vi "crane_anim_init.vi"() -> (1 "Trolley":refnum<vi>, 4 "Main":refnum<vi>(3d-picture), 5 "Pivot Beta":refnum<vi>, 6 "Arm":refnum<vi>, 7 "Load":refnum<vi>, 8 "Target":refnum<vi>, 9 "Load Line":refnum<vi>, 10 "Pivot Alpha":refnum<vi>)   [LabVIEW 2009]
uses:
  <vilib>/picture/3D Picture Control/NI_3D Picture Control.lvlib
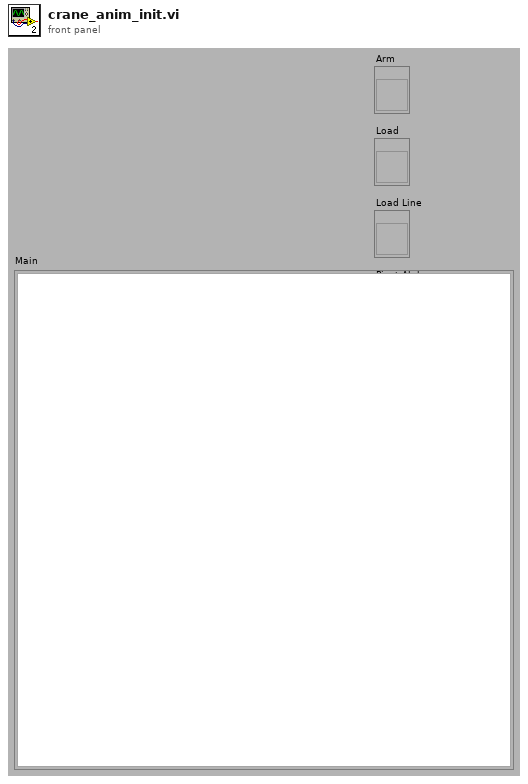
[diagram p1: front panel]
types:
  T1 = cluster{"Red":sgl, "Green":sgl, "Blue":sgl, "Alpha":sgl}
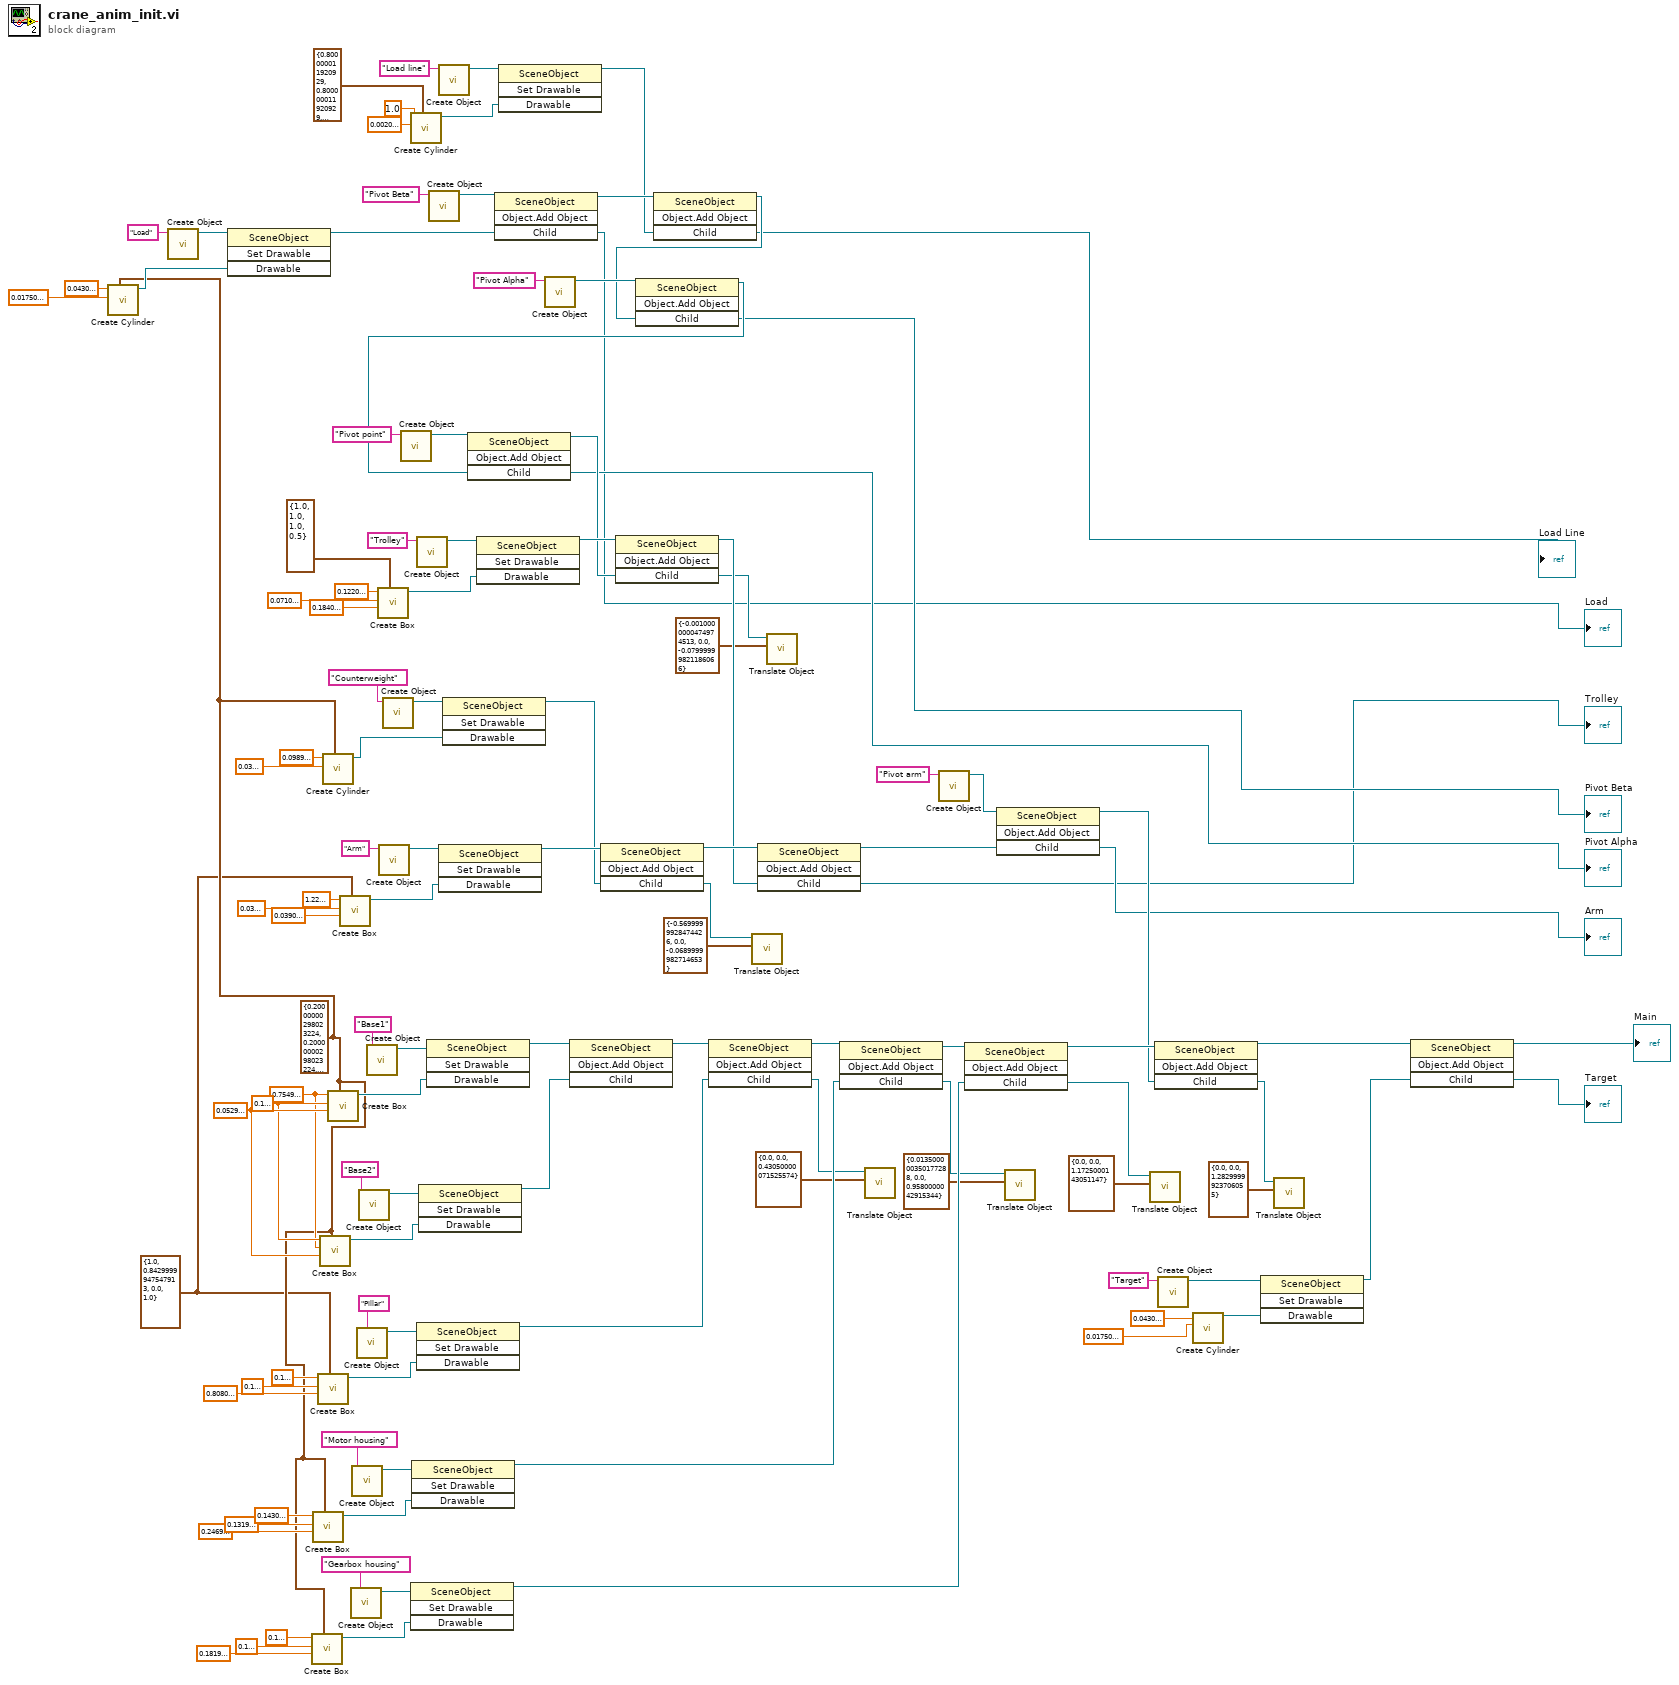
[diagram p0: block diagram]
diagram:
  w21 = T1 {"Red"=1.0, "Green"=0.843, "Blue"=0.0, "Alpha"=1.0} ("Color")
  w111 = sgl 0.053 ("Length Z")
  w110 = sgl 0.1 ("Length Y")
  w109 = sgl 0.755 ("Length X")
  w22 = T1 {"Red"=0.2, "Green"=0.2, "Blue"=0.2, "Alpha"=1.0} ("Color")
  n1 = call <vilib>:"Create Cylinder.vi"("Color"=w22, "Radius"=sgl 0.0175, "Height"=sgl 0.043) -> ("New Cylinder Refnum"=w57:refnum<vi>)  [unwired: 7 in, 1 out]
  n2 = call <vilib>:"Create Object.vi"("Name"="Load") -> ("Scene:New Object"=w58:refnum<vi>)  [unwired: 9 in, 1 out]
  n3 = invoke class="SceneObject" method="Set Drawable"(reference=w58, "Drawable"=w57) -> (reference out=w37:refnum<vi>)  [unwired: 2 in, 3 out]
  n4 = call <vilib>:"Create Box.vi"("Color"=w22, "Length Z"=sgl 0.182, "Length Y"=sgl 0.1, "Length X"=sgl 0.1) -> ("New Box Refnum"=w95:refnum<vi>)  [unwired: 6 in, 1 out]
  n5 = call <vilib>:"Create Box.vi"("Color"=w22, "Length Z"=sgl 0.247, "Length Y"=sgl 0.132, "Length X"=sgl 0.143) -> ("New Box Refnum"=w100:refnum<vi>)  [unwired: 6 in, 1 out]
  n6 = call <vilib>:"Create Box.vi"("Color"=w21, "Length Z"=sgl 0.808, "Length Y"=sgl 0.1, "Length X"=sgl 0.1) -> ("New Box Refnum"=w105:refnum<vi>)  [unwired: 6 in, 1 out]
  n7 = call <vilib>:"Create Box.vi"("Color"=w22, "Length Z"=w111, "Length Y"=w109, "Length X"=w110) -> ("New Box Refnum"=w112:refnum<vi>)  [unwired: 6 in, 1 out]
  n8 = call <vilib>:"Create Cylinder.vi"("Color"=w22, "Radius"=sgl 0.04, "Height"=sgl 0.099) -> ("New Cylinder Refnum"=w71:refnum<vi>)  [unwired: 7 in, 1 out]
  n9 = call <vilib>:"Create Box.vi"("Color"=w22, "Length Z"=w111, "Length Y"=w110, "Length X"=w109) -> ("New Box Refnum"=w114:refnum<vi>)  [unwired: 6 in, 1 out]
  n10 = call <vilib>:"Create Box.vi"("Color"=w21, "Length Z"=sgl 0.039, "Length Y"=sgl 0.04, "Length X"=sgl 1.22) -> ("New Box Refnum"=w78:refnum<vi>)  [unwired: 6 in, 1 out]
  n11 = call <vilib>:"Create Object.vi"("Name"="Gearbox housing") -> ("Scene:New Object"=w96:refnum<vi>)  [unwired: 9 in, 1 out]
  n12 = call <vilib>:"Create Object.vi"("Name"="Motor housing") -> ("Scene:New Object"=w101:refnum<vi>)  [unwired: 9 in, 1 out]
  n13 = call <vilib>:"Create Object.vi"("Name"="Pillar") -> ("Scene:New Object"=w106:refnum<vi>)  [unwired: 9 in, 1 out]
  n14 = call <vilib>:"Create Object.vi"("Name"="Base2") -> ("Scene:New Object"=w113:refnum<vi>)  [unwired: 9 in, 1 out]
  n15 = call <vilib>:"Create Object.vi"("Name"="Base1") -> ("Scene:New Object"=w115:refnum<vi>)  [unwired: 9 in, 1 out]
  n16 = call <vilib>:"Create Box.vi"("Color"=T1 {"Red"=1.0, "Green"=1.0, "Blue"=1.0, "Alpha"=0.5}, "Length Z"=sgl 0.184, "Length Y"=sgl 0.071, "Length X"=sgl 0.122) -> ("New Box Refnum"=w62:refnum<vi>)  [unwired: 6 in, 1 out]
  n17 = call <vilib>:"Create Object.vi"("Name"="Arm") -> ("Scene:New Object"=w79:refnum<vi>)  [unwired: 9 in, 1 out]
  n18 = call <vilib>:"Create Object.vi"("Name"="Counterweight") -> ("Scene:New Object"=w72:refnum<vi>)  [unwired: 9 in, 1 out]
  n19 = call <vilib>:"Create Object.vi"("Name"="Pivot point") -> ("Scene:New Object"=w34:refnum<vi>)  [unwired: 9 in, 1 out]
  n20 = call <vilib>:"Create Cylinder.vi"("Color"=T1 {"Red"=0.8, "Green"=0.8, "Blue"=0.8, "Alpha"=1.0}, "Radius"=sgl 0.002, "Height"=sgl 1.0) -> ("New Cylinder Refnum"=w14:refnum<vi>)  [unwired: 7 in, 1 out]
  n21 = invoke class="SceneObject" method="Set Drawable"(reference=w96, "Drawable"=w95) -> (reference out=w86:refnum<vi>)  [unwired: 2 in, 3 out]
  n22 = invoke class="SceneObject" method="Set Drawable"(reference=w101, "Drawable"=w100) -> (reference out=w88:refnum<vi>)  [unwired: 2 in, 3 out]
  n23 = call <vilib>:"Create Object.vi"("Name"="Trolley") -> ("Scene:New Object"=w63:refnum<vi>)  [unwired: 9 in, 1 out]
  n24 = invoke class="SceneObject" method="Set Drawable"(reference=w106, "Drawable"=w105) -> (reference out=w89:refnum<vi>)  [unwired: 2 in, 3 out]
  n25 = invoke class="SceneObject" method="Set Drawable"(reference=w113, "Drawable"=w112) -> (reference out=w107:refnum<vi>)  [unwired: 2 in, 3 out]
  n26 = invoke class="SceneObject" method="Set Drawable"(reference=w115, "Drawable"=w114) -> (reference out=w108:refnum<vi>)  [unwired: 2 in, 3 out]
  n27 = call <vilib>:"Create Object.vi"("Name"="Pivot Beta") -> ("Scene:New Object"=w39:refnum<vi>)  [unwired: 9 in, 1 out]
  n28 = call <vilib>:"Create Object.vi"("Name"="Load line") -> ("Scene:New Object"=w16:refnum<vi>)  [unwired: 9 in, 1 out]
  n29 = invoke class="SceneObject" method="Set Drawable"(reference=w79, "Drawable"=w78) -> (reference out=w68:refnum<vi>)  [unwired: 2 in, 3 out]
  n30 = invoke class="SceneObject" method="Set Drawable"(reference=w72, "Drawable"=w71) -> (reference out=w67:refnum<vi>)  [unwired: 2 in, 3 out]
  n31 = invoke class="SceneObject" method="Set Drawable"(reference=w63, "Drawable"=w62) -> (reference out=w53:refnum<vi>)  [unwired: 2 in, 3 out]
  n32 = invoke class="SceneObject" method="Object.Add Object"(reference=w39, "Child"=w37) -> (reference out=w19:refnum<vi>, "Child"=→"Load":refnum<vi>)  [unwired: 2 in, 2 out]
  n33 = invoke class="SceneObject" method="Set Drawable"(reference=w16, "Drawable"=w14) -> (reference out=w17:refnum<vi>)  [unwired: 2 in, 3 out]
  n34 = call <vilib>:"Create Object.vi"("Name"="Pivot Alpha") -> ("Scene:New Object"=w52:refnum<vi>)  [unwired: 9 in, 1 out]
  n35 = invoke class="SceneObject" method="Object.Add Object"(reference=w108, "Child"=w107) -> (reference out=w91:refnum<vi>)  [unwired: 2 in, 3 out]
  n36 = invoke class="SceneObject" method="Object.Add Object"(reference=w68, "Child"=w67) -> (reference out=w64:refnum<vi>, "Child"=w66:refnum<vi>)  [unwired: 2 in, 2 out]
  n37 = invoke class="SceneObject" method="Object.Add Object"(reference=w19, "Child"=w17) -> (reference out=w18:refnum<vi>, "Child"=→"Load Line":refnum<vi>)  [unwired: 2 in, 2 out]
  n38 = invoke class="SceneObject" method="Object.Add Object"(reference=w52, "Child"=w18) -> (reference out=w35:refnum<vi>, "Child"=→"Pivot Beta":refnum<vi>)  [unwired: 2 in, 2 out]
  n39 = invoke class="SceneObject" method="Object.Add Object"(reference=w34, "Child"=w35) -> (reference out=w36:refnum<vi>, "Child"=→"Pivot Alpha":refnum<vi>)  [unwired: 2 in, 2 out]
  n40 = invoke class="SceneObject" method="Object.Add Object"(reference=w53, "Child"=w36) -> (reference out=w54:refnum<vi>, "Child"=w50:refnum<vi>)  [unwired: 2 in, 2 out]
  n41 = invoke class="SceneObject" method="Object.Add Object"(reference=w91, "Child"=w89) -> (reference out=w90:refnum<vi>, "Child"=w85:refnum<vi>)  [unwired: 2 in, 2 out]
  n42 = call <vilib>:"Translate Object.vi"("Translation"=cluster{"X":sgl, "Y":sgl, "Z":sgl} {"X"=-0.57, "Y"=0.0, "Z"=-0.069}, "Scene.Object In"=w66) -> ()  [unwired: 8 in, 2 out]
  n43 = invoke class="SceneObject" method="Object.Add Object"(reference=w64, "Child"=w54) -> (reference out=w30:refnum<vi>, "Child"=→"Trolley":refnum<vi>)  [unwired: 2 in, 2 out]
  n44 = call <vilib>:"Translate Object.vi"("Translation"=cluster{"X":sgl, "Y":sgl, "Z":sgl} {"X"=-0.001, "Y"=0.0, "Z"=-0.08}, "Scene.Object In"=w50) -> ()  [unwired: 8 in, 2 out]
  n45 = invoke class="SceneObject" method="Object.Add Object"(reference=w90, "Child"=w88) -> (reference out=w87:refnum<vi>, "Child"=w83:refnum<vi>)  [unwired: 2 in, 2 out]
  n46 = call <vilib>:"Translate Object.vi"("Translation"=cluster{"X":sgl, "Y":sgl, "Z":sgl} {"X"=0.0, "Y"=0.0, "Z"=0.4305}, "Scene.Object In"=w85) -> ()  [unwired: 8 in, 2 out]
  n47 = call <vilib>:"Create Object.vi"("Name"="Pivot arm") -> ("Scene:New Object"=w32:refnum<vi>)  [unwired: 9 in, 1 out]
  n48 = invoke class="SceneObject" method="Object.Add Object"(reference=w87, "Child"=w86) -> (reference out=w74:refnum<vi>, "Child"=w81:refnum<vi>)  [unwired: 2 in, 2 out]
  n49 = invoke class="SceneObject" method="Object.Add Object"(reference=w32, "Child"=w30) -> (reference out=w29:refnum<vi>, "Child"=→"Arm":refnum<vi>)  [unwired: 2 in, 2 out]
  n50 = call <vilib>:"Translate Object.vi"("Translation"=cluster{"X":sgl, "Y":sgl, "Z":sgl} {"X"=0.0135, "Y"=0.0, "Z"=0.958}, "Scene.Object In"=w83) -> ()  [unwired: 8 in, 2 out]
  n51 = call <vilib>:"Translate Object.vi"("Translation"=cluster{"X":sgl, "Y":sgl, "Z":sgl} {"X"=0.0, "Y"=0.0, "Z"=1.1725}, "Scene.Object In"=w81) -> ()  [unwired: 8 in, 2 out]
  n52 = invoke class="SceneObject" method="Object.Add Object"(reference=w74, "Child"=w29) -> (reference out=w9:refnum<vi>, "Child"=w28:refnum<vi>)  [unwired: 2 in, 2 out]
  n53 = call <vilib>:"Create Object.vi"("Name"="Target") -> ("Scene:New Object"=w7:refnum<vi>)  [unwired: 9 in, 1 out]
  n54 = call <vilib>:"Create Cylinder.vi"("Radius"=sgl 0.0175, "Height"=sgl 0.043) -> ("New Cylinder Refnum"=w8:refnum<vi>)  [unwired: 8 in, 1 out]
  n55 = invoke class="SceneObject" method="Set Drawable"(reference=w7, "Drawable"=w8) -> (reference out=w3:refnum<vi>)  [unwired: 2 in, 3 out]
  n56 = call <vilib>:"Translate Object.vi"("Translation"=cluster{"X":sgl, "Y":sgl, "Z":sgl} {"X"=0.0, "Y"=0.0, "Z"=1.283}, "Scene.Object In"=w28) -> ()  [unwired: 8 in, 2 out]
  n57 = invoke class="SceneObject" method="Object.Add Object"(reference=w9, "Child"=w3) -> (reference out=→"Main":refnum<vi>, "Child"=→"Target":refnum<vi>)  [unwired: 2 in, 2 out]
